vi "Update Transfer.vi"(8 "error in (no error)":errorcluster, 9 "data":string, 10 "Transfer":refnum<class "Transfer.lvclass">, 11 "UDP Transceiver in":refnum<class "UDP Transceiver.lvclass">) -> (0 "error out":errorcluster, 3 "UDP Transceiver out":refnum<class "UDP Transceiver.lvclass">)   [LabVIEW 2017, in "UDP Transceiver.lvlib" / "UDP Transceiver.lvclass"]
uses:
  UDP Transceiver.lvclass
  Builds/Current/Data Sharing Framework Core/Data Sharing Framework Core.lvlibp/Engine/Transfer/Transfer.lvclass
  UDP Size Mismatch Error.vi
  <vilib>/NI/Static Error Handling/VIs/Static Error Handling.Source Buffer.Write.String.vi
  <vilib>/NI/Static Error Handling/VIs/Static Error Handling.Source Buffer.Write.Numeric.Scalar.Base10.vi
  <vilib>/NI/Static Error Handling/VIs/Static Error Handling.Source Buffer.Write.Numeric.Scalar.Base10 (U64).vi
  Builds/Current/Data Sharing Framework Core/Data Sharing Framework Core.lvlibp/Engine/Internal/Memory/Memory Buffer/Write 1D Array of U8.vi
  Create UDP Error.vi
  Builds/Current/Data Sharing Framework Core/Data Sharing Framework Core.lvlibp/Engine/Internal/Memory/Memory Buffer/Memory Buffer.lvclass
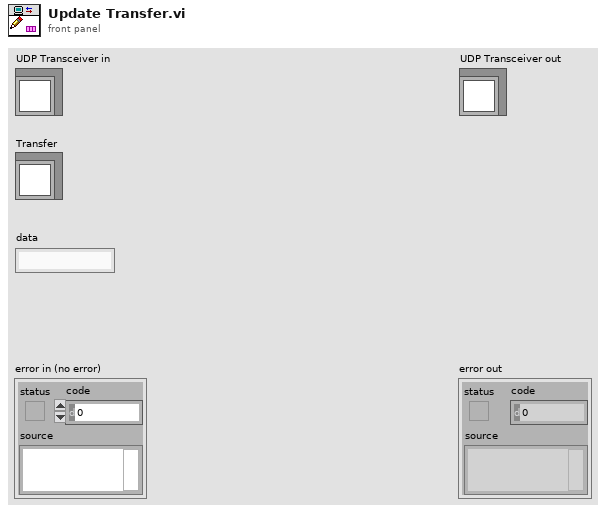
[diagram p1: front panel]
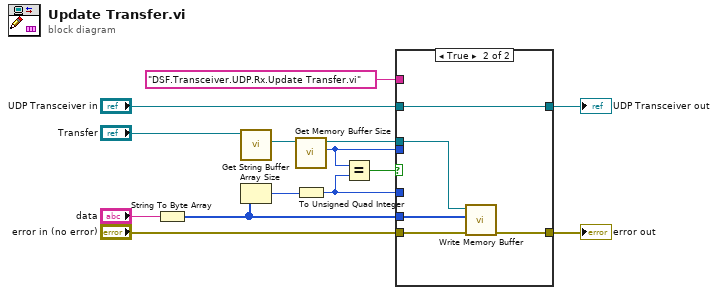
[diagram p0: block diagram]
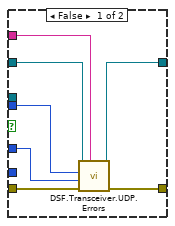
[diagram p2: hidden frame]
diagram:
  n1 = String To Byte Array(string="data") -> (unsigned byte array=w7:u8[])
  n2 = call "Get String Buffer.vi"("Transfer in"="Transfer") -> ("Buffer"=w14:refnum<class "Memory Buffer.lvclass">)  [unwired: 9 in, 1 out]
  n3 = Array Size(array=w7) -> (size(s)=w13:i32)
  n4 = call "Get Memory Buffer Size.vi"("Buffer in"=w14) -> ("buffer size"=w3:u64, "Buffer out"=w12:refnum<class "Memory Buffer.lvclass">)  [unwired: 9 in]
  n5 = To Unsigned Quad Integer(1:w13) -> (0:w2:u64)
  n6 = Equal?(x=w3, y=w2) -> (x = y?=w4:bool)
  n7 = case shown="True" w4 {
    tunnel: w12 -> [_ w26]
    tunnel: "error in (no error)" -> [w21 w25]
    tunnel: [w20 w24] -> w9
    tunnel: w7 -> [_ w22]
    tunnel: "UDP Transceiver in" -> [w19 w23]
    tunnel: [w18 w23] -> w5
    tunnel: w3 -> [w16 _]
    tunnel: w2 -> [w17 _]
    tunnel: "DSF.Transceiver.UDP.Rx.Update Transfer.vi" ("source vi name") -> [w15 _]
    frame False {
      n8 = call-poly "DSF.Transceiver.UDP.Errors.vi"("source vi name"=w15, "error in (no error)"=w21, "actual size"=w17, "expected size"=w16, "UDP Transceiver in"=w19) -> ("error out"=w20:errorcluster, "UDP Transceiver out"=w18:refnum<class "UDP Transceiver.lvclass">)  [unwired: 5 in]
    }
    frame True {
      n9 = call-poly "Write Memory Buffer.vi"("error in (no error)"=w25, "buffer in"=w22, "Buffer in"=w26) -> ("error out"=w24:errorcluster)  [unwired: 5 in, 3 out]
    }
  }
  "error out" <- w9
  "UDP Transceiver out" <- w5
